vi "Test Improve with 2d array support Recursion agains slow one.vi"() -> ()   [LabVIEW 2020, in "jki_python_data_tools.lvlib"]
uses:
  jki_python_data_tools.lvlib
panel:
  out "Array 2":i16[][](array[numeric])
  out "Speed improvement":dbl
  out "Identical String Result?":bool
  out "Iteration Time (ms) 2":dbl
  out "Iteration Time (ms)":dbl
  in  "Iteration":i32
  out "Python String":string
  out "Python String 2":string
  # "Copyright © 2003-2009 JKI. All rights reserved.\n\nAuthor: Jim Kring [jim.kring@jameskring.com]\n\nThis library is provided \"AS IS\" ,WITHOUT WARRANTIES OR \nCONDITIONS OF ANY KIND, either express or implied.\n\nJames Kring, Inc. -- http://www.jameskring.com"
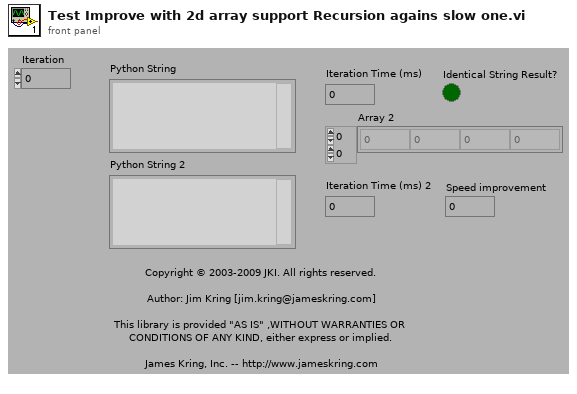
[diagram p1: front panel]
types:
  T1 = cluster{"timestamp":string, "Channel Names":string[], "Channel Data":variant}
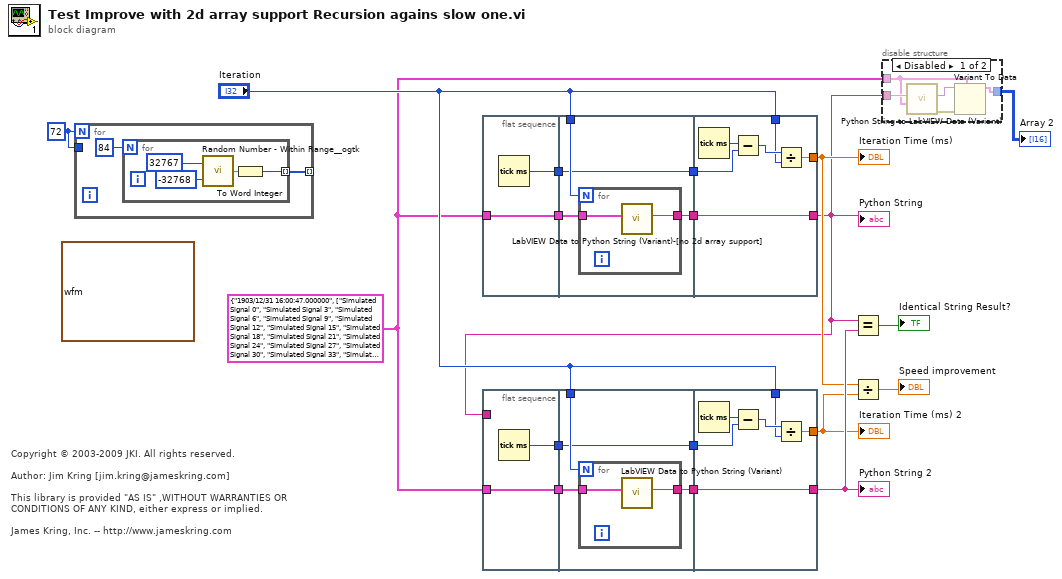
[diagram p0: block diagram]
diagram:
  w4 = 72
  w1 = T1 {"timestamp"="1903/12/31 16:00:47.000000", "Channel Names"=["Simulated Signal 0", "Simulated Signal 3", "Simulated Signal 6", "Simulated Signal 9", "Simulated Signal 12", "Simulated Signal 15", "Simulated Signal 18", "Simulated Signal 21", "Simulated Signal 24", "Simulated Signal 27", "Simulated Signal 30", "Simulated Signal 33", "Simulated Signal 36", "Simulated Signal 39", "Simulated Signal 42", "Simulated Signal 45", "Simulated Signal 1", "Simulated Signal 4", "Simulated Signal 7", "Simulated Signal 10", "Simulated Signal 13", "Simulated Signal 16", "Simulated Signal 19", "Simulated Signal 22", "Simulated Signal 25", "Simulated Signal 28", "Simulated Signal 31", "Simulated Signal 34", "Simulated Signal 37", "Simulated Signal 40", "Simulated Signal 43", "Simulated Signal 46", "Simulated Signal 2", "Simulated Signal 5", "Simulated Signal 8", "Simulated Signal 11", "Simulated Signal 14", "Simulated Signal 17", "Simulated Signal 20", "Simulated Signal 23", "Simulated Signal 26", "Simulated Signal 29", "Simulated Signal 32", "Simulated Signal 35", "Simulated Signal 38", "Simulated Signal 41", "Simulated Signal 44", "Simulated Signal 47"], "Channel Data"=variant} ("output cluster")
  (unwired) waveform(dbl)[] data[36570B] ("DAQmx.Python Raw (All CHs) []")
  # "Copyright © 2003-2009 JKI. All rights reserved.\n\nAuthor: Jim Kring [jim.kring@jameskring.com]\n\nThis library is provided \"AS IS\" ,WITHOUT WARRANTIES OR \nCONDITIONS OF ANY KIND, either express or implied.\n\nJames Kring, Inc. -- http://www.jameskring.com"
  n1 = for {
    N: w4 -> [_]
    tunnel: w4 -> [_]
    tunnel: [w20] -> _ mode=indexing
    n2 = for {
      N: 84 -> [_]
      tunnel: [w21] -> w20 mode=indexing
      n3 = call <userlib>:"Random Number - Within Range__ogtk.vi"("High (1.00)"=i16 32767, "Low (0.00)"=i16 -32768) -> ("Random Number"=w22:dbl)  [unwired: 3 in]
      n4 = To Word Integer(number=w22) -> (16bit integer=w21:i16)
    }
  }
  n5 = flat-sequence {
    tunnel: w1 -> [w26]
    tunnel: [w26] -> w18
    tunnel: [w25] -> w16
    tunnel: w18 -> [w29]
    tunnel: [w30] -> w17
    tunnel: "Iteration" -> [w28]
    tunnel: w16 -> [w27]
    tunnel: [w27] -> w15
    tunnel: [w38] -> w3
    tunnel: w17 -> [w38]
    tunnel: w15 -> [w36]
    tunnel: "Iteration" -> [w34]
    tunnel: [w33] -> w7
    frame #0 {
      n6 = Tick Count (ms)() -> (millisecond timer value=w25:u32)
    }
    frame #1 {
      n7 = for {
        N: w28 -> [_]
        tunnel: [w32] -> w30
        tunnel: w29 -> [w31]
        n8 = call "LabVIEW Data to Python String (Variant)-[no 2d array support].vi"("LabVIEW Data"=w31) -> ("Python String"=w32:string)  [unwired: 9 in, 1 out]
      }
    }
    frame #2 {
      n9 = Tick Count (ms)() -> (millisecond timer value=w37:u32)
      n10 = Subtract(x=w37, y=w36) -> (x-y=w35:u32)
      n11 = Divide(x=w35, y=w34) -> (x/y=w33:dbl)
    }
  }
  n12 = flat-sequence {
    tunnel: w1 -> [w40]
    tunnel: [w40] -> w14
    tunnel: [w39] -> w13
    tunnel: w3 -> [_]
    tunnel: w14 -> [w43]
    tunnel: [w44] -> w12
    tunnel: "Iteration" -> [w42]
    tunnel: w13 -> [w41]
    tunnel: [w41] -> w11
    tunnel: [w52] -> w9
    tunnel: w12 -> [w52]
    tunnel: w11 -> [w50]
    tunnel: "Iteration" -> [w48]
    tunnel: [w47] -> w6
    frame #0 {
      n13 = Tick Count (ms)() -> (millisecond timer value=w39:u32)
    }
    frame #1 {
      n14 = for {
        N: w42 -> [_]
        tunnel: [w46] -> w44
        tunnel: w43 -> [w45]
        n15 = call "LabVIEW Data to Python String (Variant).vi"("LabVIEW Data"=w45) -> ("Python String"=w46:string)  [unwired: 9 in, 1 out]
      }
    }
    frame #2 {
      n16 = Tick Count (ms)() -> (millisecond timer value=w51:u32)
      n17 = Subtract(x=w51, y=w50) -> (x-y=w49:u32)
      n18 = Divide(x=w49, y=w48) -> (x/y=w47:dbl)
    }
  }
  n19 = Equal?(x=w3, y=w9) -> (x = y?=→"Identical String Result?":bool)
  n20 = Divide(x=w7, y=w6) -> (x/y=→"Speed improvement":dbl)
  n21 = disable-structure shown="Disabled" {
    disable-tunnel: w3 -> [w57 _]
    disable-tunnel: w1 -> [w54 _]
    disable-tunnel: [w53 _] -> w2
    frame Disabled {
      n22 = call "Python String to LabVIEW Data (Variant).vi"("type"=w54, "Python String"=w57) -> ("error out"=w56:errorcluster, "LabVIEW Data"=w55:variant)  [unwired: 8 in]
      n23 = Variant To Data(error in=w56, type=w54, Variant=w55) -> (data=w53:T1)  [unwired: 1 out]
    }
    frame Enabled {
    }
  }
  "Array 2" <- w2
  "Python String 2" <- w9
  "Python String" <- w3
  "Iteration Time (ms)" <- w7
  "Iteration Time (ms) 2" <- w6
